vi "Linear Programming without x GE 0.vi"(0 "C":dbl[](array[numeric]), 1 "M":dbl[][](array[numeric]), 2 "B":dbl[](array[numeric])) -> (3 "maximum":dbl, 4 "X":dbl[](array[numeric]), 5 "ticks":u32, 6 "error":i32)   [LabVIEW 2023]
doc: "Linear Programming without x GE 0"
uses:
  <vilib>/gmath/NI_Gmath.lvlib
panel:
  # "c.x=max!\nm.x>=b"
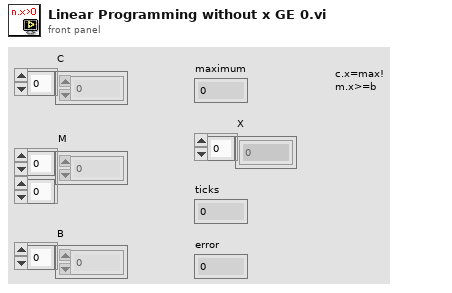
[diagram p1: front panel]
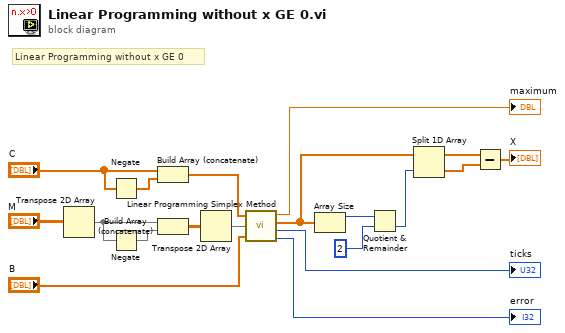
[diagram p0: block diagram]
diagram:
  # "Linear Programming without x GE 0"
  n1 = Transpose 2D Array(2D array="M") -> (transposed array=w15:dbl[][])
  n2 = Negate(x="C") -> (-x=w18:dbl[])
  n3 = Negate(x=w15) -> (-x=w17:dbl[][])
  n4 = Build Array (concatenate)("C", w18) -> (w13:dbl[])
  n5 = Build Array (concatenate)(w15, w17) -> (w14:dbl[][])
  n6 = Transpose 2D Array(2D array=w14) -> (transposed array=w2:dbl[][])
  n7 = call <vilib>:"Linear Programming Simplex Method.vi"("C"=w13, "M"=w2, "B"="B") -> ("maximum"=→"maximum":dbl, "X"=w7:dbl[], "ticks"=→"ticks":u32, "error"=→"error":i32)
  n8 = Array Size(array=w7) -> (size(s)=w8:i32)
  n9 = Quotient & Remainder(x=w8, y=2) -> (floor(x/y)=w6:i32)  [unwired: 1 out]
  n10 = Split 1D Array(array=w7, index=w6) -> (first subarray=w5:dbl[], second subarray=w3:dbl[])
  n11 = Subtract(x=w5, y=w3) -> (x-y=→"X":dbl[])
